vi "Write Wiring Cluster.vi"(8 "error in (no error)":errorcluster, 10 "Wiring Configuration":T1, 11 "Control Experiment":refnum<class "Control Experiment.lvclass">) -> (0 "error out":errorcluster, 3 "Control Experiment out":refnum<class "Control Experiment.lvclass">)   [LabVIEW 2016, in "Control Experiment.lvclass"]
uses:
  Control Experiment.lvclass
  Typedefs/Wiring Description--cluster.ctl
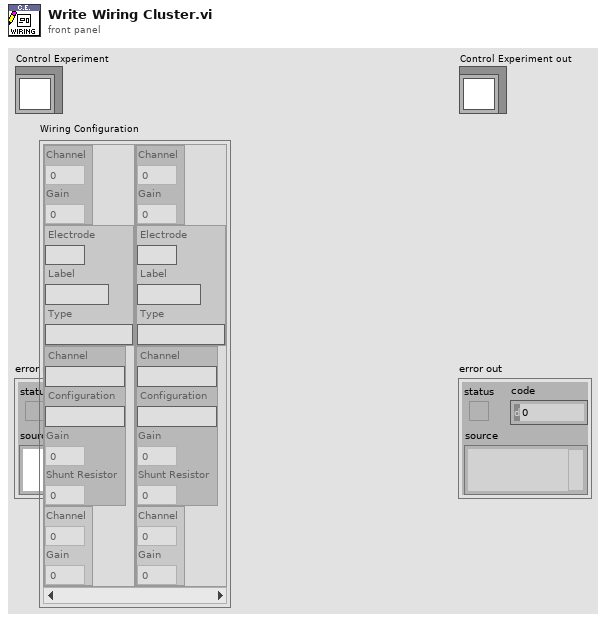
[diagram p1: front panel]
types:
  T1 = typedef "Control Experiment.lvclass/Wiring Description--cluster.ctl" = cluster{"AI":cluster{"Channel":u32, "Gain":dbl}, "Device":cluster{"Electrode":string, "Label":string, "Type":string}, "KH":cluster{"Channel":string, "Configuration":string, "Gain":u32, "Shunt Resistor":u32}, "AO":cluster{"Channel":u32, "Gain":dbl}}[]
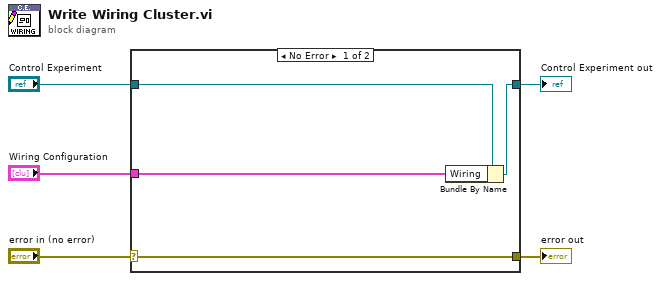
[diagram p0: block diagram]
diagram:
  n1 = case shown="No Error" "error in (no error)" {
    selector: "error in (no error)" -> [w9 w10]
    tunnel: [w9 w10] -> w4
    tunnel: [w7 w11] -> w2
    tunnel: "Control Experiment" -> [w8 w11]
    tunnel: "Wiring Configuration" -> [w6 _]
    frame No Error {
      n2 = Bundle By Name(cluster=w8, "Wiring"=w6) -> (w7:refnum<class "Control Experiment.lvclass">)
    }
    frame Error {
    }
  }
  "error out" <- w4
  "Control Experiment out" <- w2
